vi "Get General Properties.vi"(6 "Debug Build?":bool, 8 "error in (no error)":errorcluster, 10 "Build Config in":T1, 11 "Refnum in":T2) -> (0 "error out":errorcluster, 2 "Build Config out":T1, 3 "Refnum out":T2)   [LabVIEW 2019, in "PPL INI Parsing.lvlib"]
doc: "Parses the \"General\" section of the INI file to find the keys \"Description\", <>."
uses:
  PPL INI Parsing.lvlib
  <vilib>/Utility/config.llb/Config Data RefNum.ctl
  Build Configuration.ctl
  <vilib>/Utility/config.llb/Read Key (String).vi
  <vilib>/Utility/config.llb/NI_LVConfig.lvlib
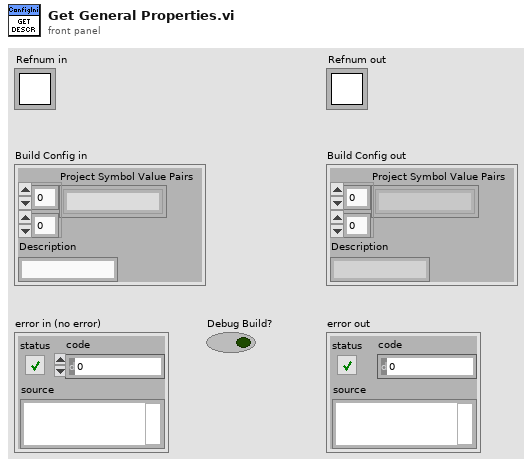
[diagram p1: front panel]
types:
  T1 = typedef "PPL INI Parsing.lvlib/Build Configuration.ctl" = cluster{"SV Pairs":string[][], "Description":string}
  T2 = typedef "NI_LVConfig.lvlib/Config Data RefNum.ctl" = refnum<k1>
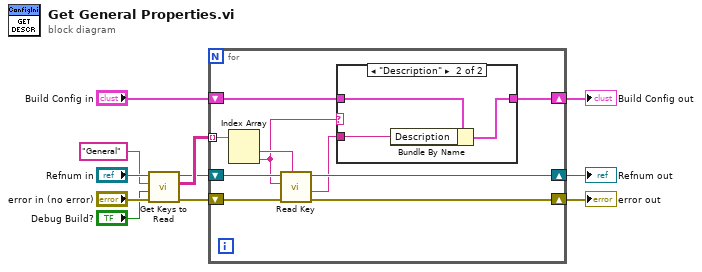
[diagram p0: block diagram]
diagram:
  n1 = call "Get Keys to Read.vi"("error in (no error)"="error in (no error)", "Debug Build?"="Debug Build?", "Section Name"="General", "Config File"="Refnum in") -> ("error out"=w9:errorcluster, "Keys to Read"=w11:string[][], "Config File"=w10:T2)  [unwired: 5 in]
  n2 = for {
    tunnel: w11 -> [w17] mode=indexing
    shift-right: [w18] -> w5
    shift-left: w10 -> [w21]
    shift-right: [w19] -> w4
    shift-left: w9 -> [w20]
    shift-right: [w12] -> w1
    shift-left: "Build Config in" -> [w13]
    n3 = Index Array(array=w17) -> (element #1=w16:string, element #2=w14:string)  [unwired: 2 in]
    n4 = call-poly <vilib>:"Read Key.vi"("section"=w16, "error in (no error)"=w20, "key"=w14, "refnum"=w21) -> ("error out"=w19:errorcluster, "value"=w15:string, "refnum out"=w18:T2)  [unwired: 4 in, 1 out]
    n5 = case shown="\"Description\"" w14 {
      tunnel: w15 -> [_ w23]
      tunnel: w13 -> [w22 w25]
      tunnel: [w22 w24] -> w12
      frame Default {
      }
      frame "Description" {
        n6 = Bundle By Name(cluster=w25, "Description"=w23) -> (w24:T1)
      }
    }
  }
  "error out" <- w4
  "Refnum out" <- w5
  "Build Config out" <- w1
